vi "Teardown Created Queues.vi"(11 "Hello World Queue in":refnum<class "Hello World Queue.lvclass">) -> (3 "Hello World Queue out":refnum<class "Hello World Queue.lvclass">)   [LabVIEW 2021, in "Hello World Queue.lvlib" / "Hello World Queue.lvclass"]
uses:
  Hello World Queue.lvclass
  Hello World Queue.lvclass/Hello World Queue.ctl
  jettl/Queue jettl/Queue jettl.lvclass
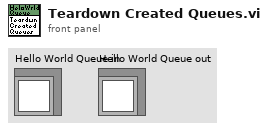
[diagram p1: front panel]
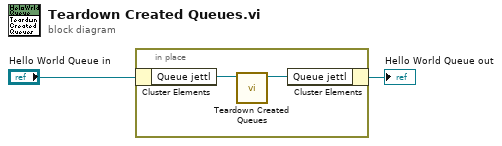
[diagram p0: block diagram]
diagram:
  n1 = in-place {
    n2 = in-place-cluster #1("Hello World Queue in") -> ("Queue jettl"=w4:refnum<class "Queue jettl.lvclass">)
    n3 = call-dynamic "Teardown Created Queues.vi"("Queue jettl in"=w4) -> ("Queue jettl out"=w3:refnum<class "Queue jettl.lvclass">)  [unwired: 10 in]
    n4 = in-place-cluster #1("Queue jettl"=w3) -> (→"Hello World Queue out":refnum<class "Hello World Queue.lvclass">)
  }
